vi "Init.vi"(5 "PathControl.lvclass":refnum<class "PathControl.lvclass">, 6 "Environmental classes":refnum<class "Instrument.lvclass">[](array[class]), 7 "XML Handler.lvclass":refnum<class "XML Handler.lvclass">, 8 "error in (no error)":errorcluster, 9 "Instruments to Use":T1(array[cluster]), 10 "Device.lvclass":refnum<class "Device.lvclass">, 11 "Harmonics in":refnum<class "Harmonics.lvclass">) -> (0 "error out":errorcluster, 3 "Harmonics out":refnum<class "Harmonics.lvclass">)   [LabVIEW 2020, in "Harmonics.lvclass"]
doc: "Initializes the measurement.\nThis verifies that the instruments are present and adds them into the class data.\nIs also adds the xml handler into the class data."
uses:
  Harmonics.lvclass
  Devices/Device.lvclass
  Instruments/Instrument.lvclass
  XML Handler/XML Handler.lvclass
  Path Control/PathControl.lvclass
  Controls/Init states.ctl
  Instruments/Spectrum Analyzer/Spectrum Analyzer.lvclass
  Instruments/Signal Generator/Signal Generator.lvclass
  Harmonics.lvclass/Harmonics.ctl
  Instruments/Power Meter/Power Meter.lvclass
  Measurement.lvclass
panel:
  out "Current State":string
  out "Initializing Harmonic Measurement":u8(slide) scale=0.0..100.0
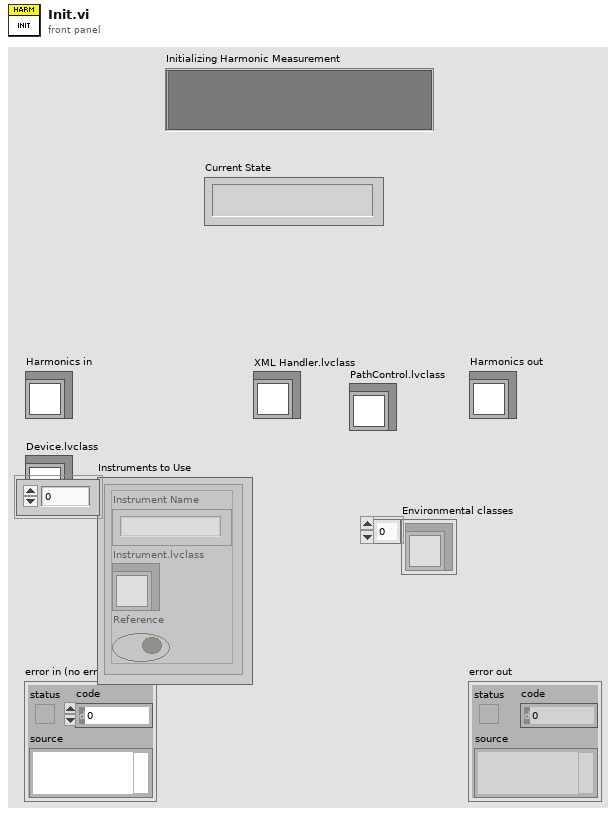
[diagram p1: front panel]
types:
  T1 = cluster{"Instrument Name":string, "Instrument.lvclass":refnum<class "Instrument.lvclass">, "Reference":bool}[]
  T2 = typedef "Harmonics.lvclass/Init states.ctl" = enum16{"Verify instruments", "Init Sweep Parameters", "Init Instruments", "Done"}
  T3 = typedef "Harmonics.lvclass/Config info.ctl" = cluster{"RBW":dbl, "VBW ":dbl, "Number of Averages":i32, "Average On":bool, "Symbols":i32[], "All Harm":bool, "Loop order":T4, "Power Window":dbl, "Frequency (MHz)":string, "Power (dBm)":string, "PM for power leveling":u8, "Zero span":bool, "Stop level":dbl}
  T4 = typedef "Harmonics.lvclass/Loop order.ctl" = enum16{"Device -> Power -> Frequency", "Device -> Frequency -> Power"}
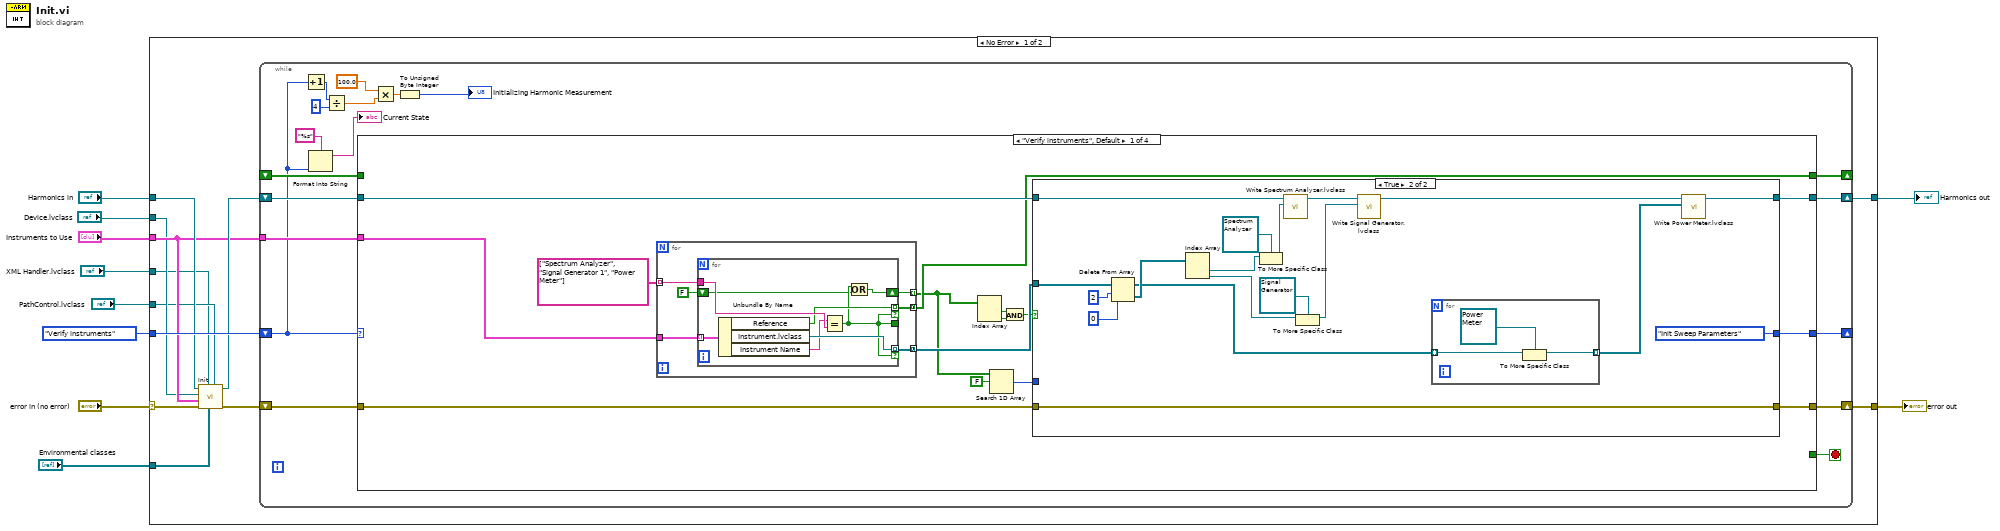
[diagram p0: block diagram]
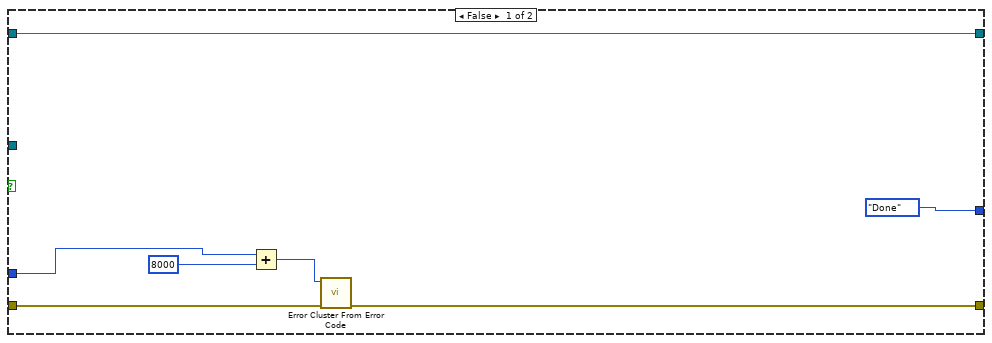
[diagram p2: hidden frame]
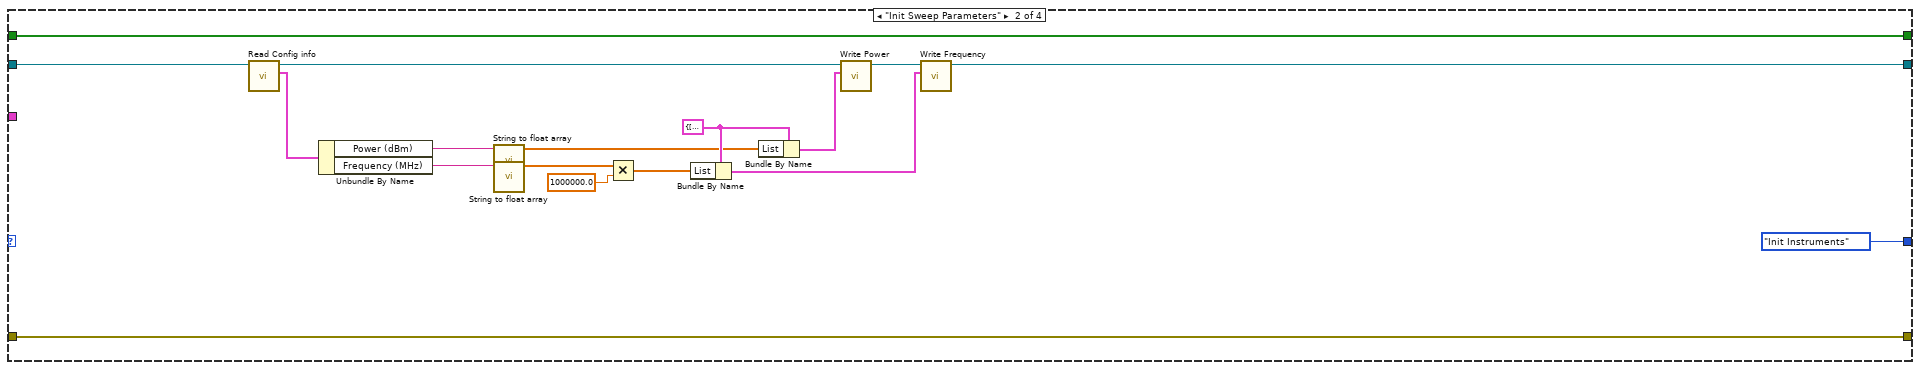
[diagram p3: hidden frame]
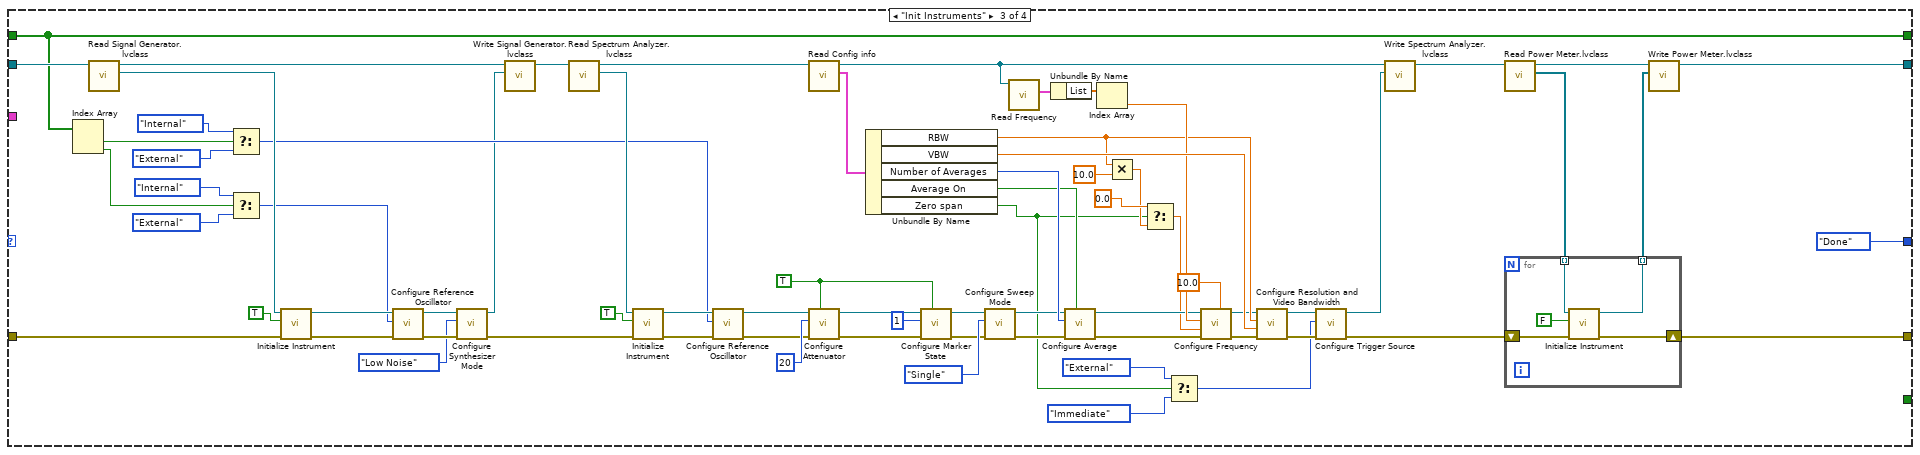
[diagram p4: hidden frame]
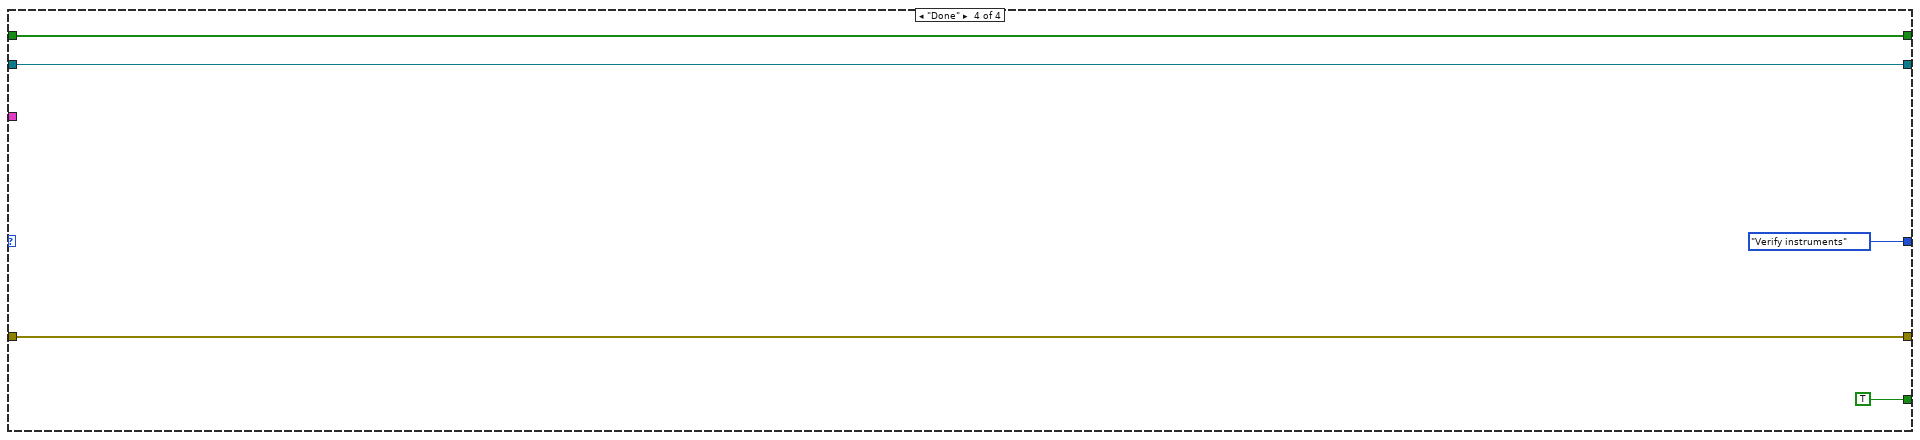
[diagram p5: hidden frame]
diagram:
  n1 = case shown="No Error" "error in (no error)" {
    selector: "error in (no error)" -> [w17 w197]
    tunnel: "Instruments to Use" -> [w15 _]
    tunnel: "Device.lvclass" -> [w14 _]
    tunnel: "Harmonics in" -> [w19 w198]
    tunnel: Init_states."Verify instruments" -> [w22 _]
    tunnel: [w21 w197] -> w5
    tunnel: [w20 w198] -> w4
    tunnel: "XML Handler.lvclass" -> [w12 _]
    tunnel: "PathControl.lvclass" -> [w13 _]
    tunnel: "Environmental classes" -> [w11 _]
    frame No Error {
      n2 = call-parent "Init.vi"("PathControl.lvclass"=w13, "Environmental classes"=w11, "XML Handler.lvclass"=w12, "error in (no error)"=w17, "Instruments to Use"=w15, "Device.lvclass"=w14, "Measurements in"=w19) -> ("error out"=w16:errorcluster, "Measurements out"=w18:refnum<class "Harmonics.lvclass">)  [unwired: 3 in]
      n3 = while {
        shift-right: [w36] -> w21
        shift-left: w16 -> [w37]
        tunnel: w15 -> [w40]
        shift-right: [w38] -> w20
        shift-left: w18 -> [w39]
        shift-right: [w34] -> _
        shift-left: w22 -> [w29]
        shift-right: [w33] -> _
        shift-left: _ -> [w32]
        stop <- w35 stop-if-true
        n4 = Increment(x=w29) -> (x+1=w28:T2)
        n5 = Format Into String(format string="%s", w29) -> (resulting string=→"Current State":string)  [unwired: 2 in, 1 out]
        n6 = Divide(x=w28, y=4) -> (x/y=w26:dbl)
        n7 = case shown="\"Verify instruments\", Default" w29 {
          tunnel: w40 -> [w49 _ _ _]
          tunnel: w39 -> [w52 w112 w186 w192]
          tunnel: [w55 w108 w137 w192] -> w38
          tunnel: w37 -> [w51 w113 w183 w194]
          tunnel: [w54 w113 w136 w194] -> w36
          tunnel: [w53 Init_states."Init Instruments" Init_states."Done" Init_states."Verify instruments"] -> w34
          tunnel: [_ _ _ TRUE] -> w35
          tunnel: [w44 w104 w164 w196] -> w33
          tunnel: w32 -> [_ w104 w164 w196]
          frame "Verify instruments", Default {
            n8 = for {
              tunnel: [w61] -> w48 mode=concatenating
              tunnel: [w56] -> w43 mode=indexing
              tunnel: [w60] -> w44 mode=concatenating
              tunnel: string[] ["Spectrum Analyzer", "Signal Generator 1", "Power Meter"] -> [w59] mode=indexing
              tunnel: w49 -> [w58]
              n9 = for {
                tunnel: w58 -> [w66] mode=indexing
                tunnel: w59 -> [w69]
                tunnel: [w68] -> w61 mode=indexing if=w63
                tunnel: [w63] -> _
                tunnel: [w67] -> w60 mode=indexing if=w63
                shift-right: [w64] -> w56
                shift-left: FALSE -> [w62]
                n10 = Unbundle By Name(w66) -> ("Reference"=w67:bool, "Instrument.lvclass"=w68:refnum<class "Instrument.lvclass">, "Instrument Name"=w65:string)
                n11 = Equal?(x=w65, y=w69) -> (x = y?=w63:bool)
                n12 = Or(x=w63, y=w62) -> (x .or. y?=w64:bool)
              }
            }
            n13 = Index Array(array=w43) -> (element #1=w47:bool, element #2=w46:bool)  [unwired: 2 in]
            n14 = Search 1D Array(1D array=w43, element=FALSE) -> (index of element=w41:i32)  [unwired: 1 in]
            n15 = And(x=w47, y=w46) -> (x .and. y?=w45:bool)
            n16 = case shown="True" w45 {
              tunnel: w48 -> [_ w79]
              tunnel: w52 -> [w76 w94]
              tunnel: [w76 w83] -> w55
              tunnel: w51 -> [w75 w85]
              tunnel: [w72 w85] -> w54
              tunnel: [Init_states."Done" Init_states."Init Sweep Parameters"] -> w53
              tunnel: w41 -> [w70 _]
              frame False {
                n17 = Add(x=w70, y=8000) -> (x+y=w73:i32)
                n18 = call <vilib>:"Error Cluster From Error Code.vi"("error in (no error)"=w75, "error code (0)"=w73) -> ("error out"=w72:errorcluster)  [unwired: 7 in]
              }
              frame True {
                n19 = Delete From Array(array=w79, length=2, index=0) -> (deleted portion=w78:refnum<class "Instrument.lvclass">[], array with subset deleted=w77:refnum<class "Instrument.lvclass">[])
                n20 = Index Array(array=w78) -> (element #1=w92:refnum<class "Instrument.lvclass">, element #2=w89:refnum<class "Instrument.lvclass">)  [unwired: 2 in]
                n21 = To More Specific Class(target class=refnum<class "Spectrum Analyzer.lvclass"> refnum ("Spectrum Analyzer.lvclass"), reference=w92) -> (specific class reference=w91:refnum<class "Spectrum Analyzer.lvclass">)  [unwired: 1 in, 1 out]
                n22 = call "Write Spectrum Analyzer.lvclass.vi"("Spectrum Analyzer.lvclass"=w91, "Harmonics in"=w94) -> ("Harmonics out"=w93:refnum<class "Harmonics.lvclass">)  [unwired: 9 in]
                n23 = To More Specific Class(target class=refnum<class "Signal Generator.lvclass"> refnum ("Signal Generator.lvclass"), reference=w89) -> (specific class reference=w87:refnum<class "Signal Generator.lvclass">)  [unwired: 1 in, 1 out]
                n24 = call "Write Signal Generator.lvclass.vi"("Signal Generator.lvclass"=w87, "Harmonics in"=w93) -> ("Harmonics out"=w84:refnum<class "Harmonics.lvclass">)  [unwired: 9 in]
                n25 = for {
                  tunnel: [w96] -> w82 mode=indexing
                  tunnel: w77 -> [w95] mode=indexing
                  n26 = To More Specific Class(target class=refnum<class "Power Meter.lvclass"> refnum ("Power Meter.lvclass"), reference=w95) -> (specific class reference=w96:refnum<class "Power Meter.lvclass">)  [unwired: 1 in, 1 out]
                }
                n27 = call "Write Power Meter.lvclass.vi"("Power Meter classes"=w82, "Harmonics in"=w84) -> ("Harmonics out"=w83:refnum<class "Harmonics.lvclass">)  [unwired: 9 in]
              }
            }
          }
          frame "Init Sweep Parameters" {
            w107 = cluster{"List":dbl[], "Index":i32, "Last":bool} {"List"=[], "Index"=0, "Last"=FALSE} ("Power")
            n28 = call "Read Config info.vi"("Harmonics in"=w112) -> ("Config info"=w111:T3, "Harmonics out"=w110:refnum<class "Harmonics.lvclass">)  [unwired: 9 in]
            n29 = Unbundle By Name(w111) -> ("Power (dBm)"=w101:string, "Frequency (MHz)"=w99:string)
            n30 = call "String to float array.vi"("String"=w101) -> ("Array - Numeric"=w100:dbl[])  [unwired: 9 in, 1 out]
            n31 = call "String to float array.vi"("String"=w99) -> ("Array - Numeric"=w103:dbl[])  [unwired: 9 in, 1 out]
            n32 = Multiply(x=w103, y=1000000.0) -> (x*y=w98:dbl[])
            n33 = Bundle By Name(cluster=w107, "List"=w98) -> (w105:cluster{"List":dbl[], "Index":i32, "Last":bool})
            n34 = Bundle By Name(cluster=w107, "List"=w100) -> (w106:cluster{"List":dbl[], "Index":i32, "Last":bool})
            n35 = call "Write Power.vi"("Power"=w106, "Harmonics in"=w110) -> ("Harmonics out"=w109:refnum<class "Harmonics.lvclass">)  [unwired: 9 in]
            n36 = call "Write Frequency.vi"("Frequency"=w105, "Harmonics in"=w109) -> ("Harmonics out"=w108:refnum<class "Harmonics.lvclass">)  [unwired: 9 in]
          }
          frame "Init Instruments" {
            w169 = TRUE ("Auto Attenuator (T)")
            n37 = Index Array(array=w164) -> (element #1=w145:bool, element #2=w146:bool)  [unwired: 2 in]
            n38 = call "Read Signal Generator.lvclass.vi"("Harmonics in"=w186) -> ("Signal Generator.lvclass"=w185:refnum<class "Signal Generator.lvclass">, "Harmonics out"=w182:refnum<class "Harmonics.lvclass">)  [unwired: 9 in]
            n39 = Select(t=enum16{"Internal", "External"}."Internal" ("Reference Mode"), s=w145, f=enum16{"Internal", "External"}."External") -> (s? t:f=w149:enum16{"Internal", "External"})
            n40 = Select(t=enum16{"Internal", "External"}."Internal" ("Reference Mode"), s=w146, f=enum16{"Internal", "External"}."External") -> (s? t:f=w160:enum16{"Internal", "External"})
            n41 = call-dynamic "Initialize Instrument.vi"("error in (no error)"=w183, "Reset"=TRUE, "Instrument in"=w185) -> ("error out"=w158:errorcluster, "Instrument out"=w163:refnum<class "Signal Generator.lvclass">)  [unwired: 7 in]
            n42 = call-dynamic "Configure Reference Oscillator.vi"("error in (no error)"=w158, "Reference Mode"=w160, "Signal Generator in"=w163) -> ("error out"=w159:errorcluster, "Signal Generator out"=w157:refnum<class "Signal Generator.lvclass">)  [unwired: 7 in]
            n43 = call-dynamic "Configure Synthesizer Mode.vi"("error in (no error)"=w159, "Synthesizer Mode"=enum16{"Normal", "Low Noise"}."Low Noise", "Signal Generator in"=w157) -> ("error out"=w155:errorcluster, "Signal Generator out"=w147:refnum<class "Signal Generator.lvclass">)  [unwired: 7 in]
            n44 = call "Write Signal Generator.lvclass.vi"("Signal Generator.lvclass"=w147, "Harmonics in"=w182) -> ("Harmonics out"=w181:refnum<class "Harmonics.lvclass">)  [unwired: 9 in]
            n45 = call "Read Spectrum Analyzer.lvclass.vi"("Harmonics in"=w181) -> ("Spectrum Analyzer.lvclass"=w180:refnum<class "Spectrum Analyzer.lvclass">, "Harmonics out"=w176:refnum<class "Harmonics.lvclass">)  [unwired: 9 in]
            n46 = call-dynamic "Initialize Instrument.vi"("error in (no error)"=w155, "Reset"=TRUE, "Instrument in"=w180) -> ("error out"=w154:errorcluster, "Instrument out"=w153:refnum<class "Spectrum Analyzer.lvclass">)  [unwired: 7 in]
            n47 = call-dynamic "Configure Reference Oscillator.vi"("error in (no error)"=w154, "Reference Oscillator (Internal)"=w149, "Spectrum Analyzer in"=w153) -> ("error out"=w151:errorcluster, "Spectrum Analyzer out"=w152:refnum<class "Spectrum Analyzer.lvclass">)  [unwired: 7 in]
            n48 = call "Read Config info.vi"("Harmonics in"=w176) -> ("Config info"=w175:T3, "Harmonics out"=w144:refnum<class "Harmonics.lvclass">)  [unwired: 9 in]
            n49 = call-dynamic "Configure Attenuator.vi"("Auto Attenuator (T)"=w169, "error in (no error)"=w151, "Attenuator (dB)"=u32 20, "Spectrum Analyzer in"=w152) -> ("error out"=w171:errorcluster, "Spectrum Analyzer out"=w170:refnum<class "Spectrum Analyzer.lvclass">)  [unwired: 6 in]
            n50 = Unbundle By Name(w175) -> ("RBW"=w140:dbl, "VBW"=w174:dbl, "Number of Averages"=w173:i32, "Average On"=w172:bool, "Zero span"=w121:bool)
            n51 = call-dynamic "Configure Marker State.vi"("Maker On (F)"=w169, "error in (no error)"=w171, "Marker Number (1)"=u32 1, "Spectrum Analyzer in"=w170) -> ("error out"=w165:errorcluster, "Spectrum Analyzer out"=w166:refnum<class "Spectrum Analyzer.lvclass">)  [unwired: 6 in]
            n52 = call-dynamic "Configure Sweep Mode.vi"("error in (no error)"=w165, "Sweep Mode"=enum16{"Continuous", "Single"}."Single", "Spectrum Analyzer in"=w166) -> ("error out"=w134:errorcluster, "Spectrum Analyzer out"=w135:refnum<class "Spectrum Analyzer.lvclass">)  [unwired: 7 in]
            n53 = call "Read Frequency.vi"("Harmonics in"=w144) -> ("Frequency"=w143:cluster{"List":dbl[], "Index":i32, "Last":bool})  [unwired: 9 in, 1 out]
            n54 = Unbundle By Name(w143) -> ("List"=w142:dbl[])
            n55 = call-dynamic "Configure Average.vi"("Average On (F)"=w172, "error in (no error)"=w134, "Average"=w173, "Spectrum Analyzer in"=w135) -> ("error out"=w133:errorcluster, "Spectrum Analyzer out"=w131:refnum<class "Spectrum Analyzer.lvclass">)  [unwired: 6 in]
            n56 = Index Array(array=w142) -> (element=w141:dbl)  [unwired: 1 in]
            n57 = Multiply(x=w140, y=10.0) -> (x*y=w128:dbl)
            n58 = Select(t=0.0 ("y"), s=w121, f=w128) -> (s? t:f=w127:dbl)
            n59 = Select(t=enum16{"Immediate", "External"}."External" ("Trigger Source"), s=w121, f=enum16{"Immediate", "External"}."Immediate" ("Trigger Source")) -> (s? t:f=w119:enum16{"Immediate", "External"})
            n60 = call-dynamic "Configure Frequency.vi"("Sweep time (ms)"=10.0, "error in (no error)"=w133, "Span/Stop Frequency [Hz]"=w127, "Center/Start Frequency [Hz]"=w141, "Spectrum Analyzer in"=w131) -> ("error out"=w132:errorcluster, "Spectrum Analyzer out"=w130:refnum<class "Spectrum Analyzer.lvclass">)  [unwired: 5 in]
            n61 = call-dynamic "Configure Resolution and Video Bandwidth.vi"("error in (no error)"=w132, "VBW [Hz]"=w174, "RBW [Hz]"=w140, "Spectrum Analyzer in"=w130) -> ("error out"=w125:errorcluster, "Spectrum Analyzer out"=w124:refnum<class "Spectrum Analyzer.lvclass">)  [unwired: 6 in]
            n62 = call-dynamic "Configure Trigger Source.vi"("error in (no error)"=w125, "Trigger Source"=w119, "Spectrum Analyzer in"=w124) -> ("error out"=w122:errorcluster, "Spectrum Analyzer out"=w123:refnum<class "Spectrum Analyzer.lvclass">)  [unwired: 7 in]
            n63 = call "Write Spectrum Analyzer.lvclass.vi"("Spectrum Analyzer.lvclass"=w123, "Harmonics in"=w144) -> ("Harmonics out"=w138:refnum<class "Harmonics.lvclass">)  [unwired: 9 in]
            n64 = call "Read Power Meter.lvclass.vi"("Harmonics in"=w138) -> ("Power Meter classes"=w117:refnum<class "Power Meter.lvclass">[], "Harmonics out"=w116:refnum<class "Harmonics.lvclass">)  [unwired: 9 in]
            n65 = for {
              tunnel: w117 -> [w190] mode=indexing
              tunnel: [w187] -> w115 mode=indexing
              shift-right: [w188] -> w136
              shift-left: w122 -> [w191]
              n66 = call-dynamic "Initialize Instrument.vi"("error in (no error)"=w191, "Reset"=FALSE, "Instrument in"=w190) -> ("error out"=w188:errorcluster, "Instrument out"=w187:refnum<class "Power Meter.lvclass">)  [unwired: 7 in]
            }
            n67 = call "Write Power Meter.lvclass.vi"("Power Meter classes"=w115, "Harmonics in"=w116) -> ("Harmonics out"=w137:refnum<class "Harmonics.lvclass">)  [unwired: 9 in]
          }
          frame "Done" {
          }
        }
        n68 = Multiply(x=100.0 ("y"), y=w26) -> (x*y=w24:dbl)
        n69 = To Unsigned Byte Integer(number=w24) -> (unsigned 8bit integer=→"Initializing Harmonic Measurement":u8)
      }
    }
    frame Error {
    }
  }
  "error out" <- w5
  "Harmonics out" <- w4
